vi "40G RF Switch Tool(NI 6509).vi"(4 "error in":errorcluster, 5 "Index":i8 min=0 max=100, 6 "arrayinput(1-48)":bool[][](array[boolean]), 7 "DAQ Device":enum16{"Dev1", "Dev2", "Dev3"}(ring)) -> ()   [LabVIEW 2011]
uses:
  <vilib>/Utility/error.llb/DialogType.ctl
  <vilib>/Utility/file.llb/Read From Spreadsheet File (I64).vi
  <vilib>/Utility/file.llb/Write To Spreadsheet File (I64).vi
panel:
  in  "Arrayinput":bool[][](array[boolean])=array80x96[7680 elements]
  in  "Tap":enum32{"P1-P5", "P6-P11"}(tab)
  in  "Index 3":i32[](array[numeric])=[1, 2, 3, 4, 5, 6, 7, 8, 9, 10, 11, 12, 13, 14, 15, 16, 17, 18, 19, 20, 21, 22, 23, 24, 25, 26, 27, 28, 29, 30, 31, 32, 33, 34, 35, 36, 37, 38, 39, 40, 41, 42, 43, 44, 45, 46, 47, 48, 49, 50, 51, 52, 53, 54, 55, 56, 57, 58, 59, 60, 61, 62, 63, 64, 65, 66, 67, 68, 69, 70, 71, 72, 73, 74, 75, 76, 77, 78, 79, 80]
  in  "PCI-6509: P0-P1-P2-P3-P4-P5":dbl[](array[numeric])=[0.0, 1.0, 2.0, 3.0, 4.0, 5.0, 6.0, 7.0, 0.0, 1.0, 2.0, 3.0, 4.0, 5.0, 6.0, 7.0, 0.0, 1.0, 2.0, 3.0, 4.0, 5.0, 6.0, 7.0, 0.0, 1.0, 2.0, 3.0, 4.0, 5.0, 6.0, 7.0, 0.0, 1.0, 2.0, 3.0, 4.0, 5.0, 6.0, 7.0, 0.0, 1.0, 2.0, 3.0, 4.0, 5.0, 6.0, 7.0]
  in  "Index 2":i32[](array[numeric])=[1, 2, 3, 4, 5, 6, 7, 8, 9, 10, 11, 12, 13, 14, 15, 16, 17, 18, 19, 20, 21, 22, 23, 24, 25, 26, 27, 28, 29, 30, 31, 32, 33, 34, 35, 36, 37, 38, 39, 40, 41, 42, 43, 44, 45, 46, 47, 48, 49, 50, 51, 52, 53, 54, 55, 56, 57, 58, 59, 60, 61, 62, 63, 64, 65, 66, 67, 68, 69, 70, 71, 72, 73, 74, 75, 76, 77, 78, 79, 80]
  in  "PCI-6509: P6-P7-P8-P9-P10-P11":dbl[](array[numeric])=[0.0, 1.0, 2.0, 3.0, 4.0, 5.0, 6.0, 7.0, 0.0, 1.0, 2.0, 3.0, 4.0, 5.0, 6.0, 7.0, 0.0, 1.0, 2.0, 3.0, 4.0, 5.0, 6.0, 7.0, 0.0, 1.0, 2.0, 3.0, 4.0, 5.0, 6.0, 7.0, 0.0, 1.0, 2.0, 3.0, 4.0, 5.0, 6.0, 7.0, 0.0, 1.0, 2.0, 3.0, 4.0, 5.0, 6.0, 7.0]
  in  "array input (49~96)":bool[][](array[boolean])
  in  "Switch Matrix":u16(ring)=4
  in  "Basic Path":path=path "D:/HPTS Development/VNA Automatic Data Save Tool 20151010(No DAQ)/Switch Matrix"
  out "Matrix List":string[](array[string])
  out "Path":path=path "D:/HPTS Development/VNA Automatic Data Save Tool 20151010(No DAQ)/Switch Matrix"
  in  "Modify":bool
  in  "Lines 4":tag="Dev3/port0/line0:7, Dev3/port1/line0:7, Dev3/port2/line0:7, Dev3/port3/line0:7, Dev3/port4/line0:7, Dev3/port5/line0:7, Dev3/port6/line0:7, Dev3/port7/line0:7, Dev3/port8/line0:7, Dev3/port9/line0:7, Dev3/port10/line0:7, Dev3/port11/line0:7" caption="Lines"
  in  "Lines 2":tag="Dev2/port0/line0:7, Dev2/port1/line0:7, Dev2/port2/line0:7, Dev2/port3/line0:7, Dev2/port4/line0:7, Dev2/port5/line0:7, Dev2/port6/line0:7, Dev2/port7/line0:7, Dev2/port8/line0:7, Dev2/port9/line0:7, Dev2/port10/line0:7, Dev2/port11/line0:7" caption="Lines"
  in  "Lines":tag="Dev1/port0/line0:7, Dev1/port1/line0:7, Dev1/port2/line0:7, Dev1/port3/line0:7, Dev1/port4/line0:7, Dev1/port5/line0:7, Dev1/port6/line0:7, Dev1/port7/line0:7, Dev1/port8/line0:7, Dev1/port9/line0:7, Dev1/port10/line0:7, Dev1/port11/line0:7"
  in  "name to assign":string="NI6509"
  # "RF Matrix Control System By NI PCI-6509 DAQmx Card"
  # "20151016"
  # "SW-04 A"
  # "SW01 & 02"
  # "SW-02 A"
  # "SW-03 A"
  # "SW-01 A"
  # "-------------P0------------"
  # "-------------P1------------"
  # "-------------P2------------"
  # "-------------P3------------"
  # "-------------P4------------"
  # "-------------P5------------"
  # "SW-01 B"
  # "SW-04 B"
  # "SW03 & SW04"
  # "SW-02 B"
  # "SW-03 B"
  # "-------------P6------------"
  # "-------------P7------------"
  # "-------------P8------------"
  # "------------P9------------"
  # "-------------P10----------"
  # "-------------P11-----------"
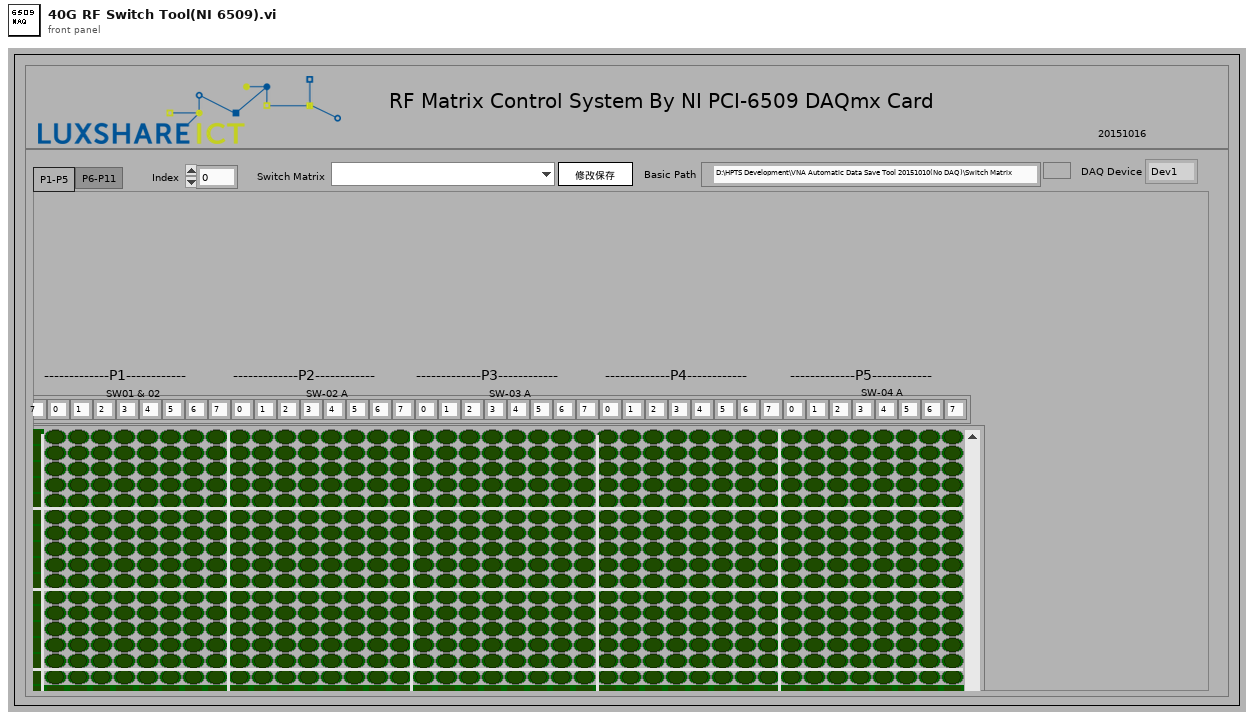
[diagram p1: front panel]
types:
  T1 = typedef "DialogType.ctl" = u16
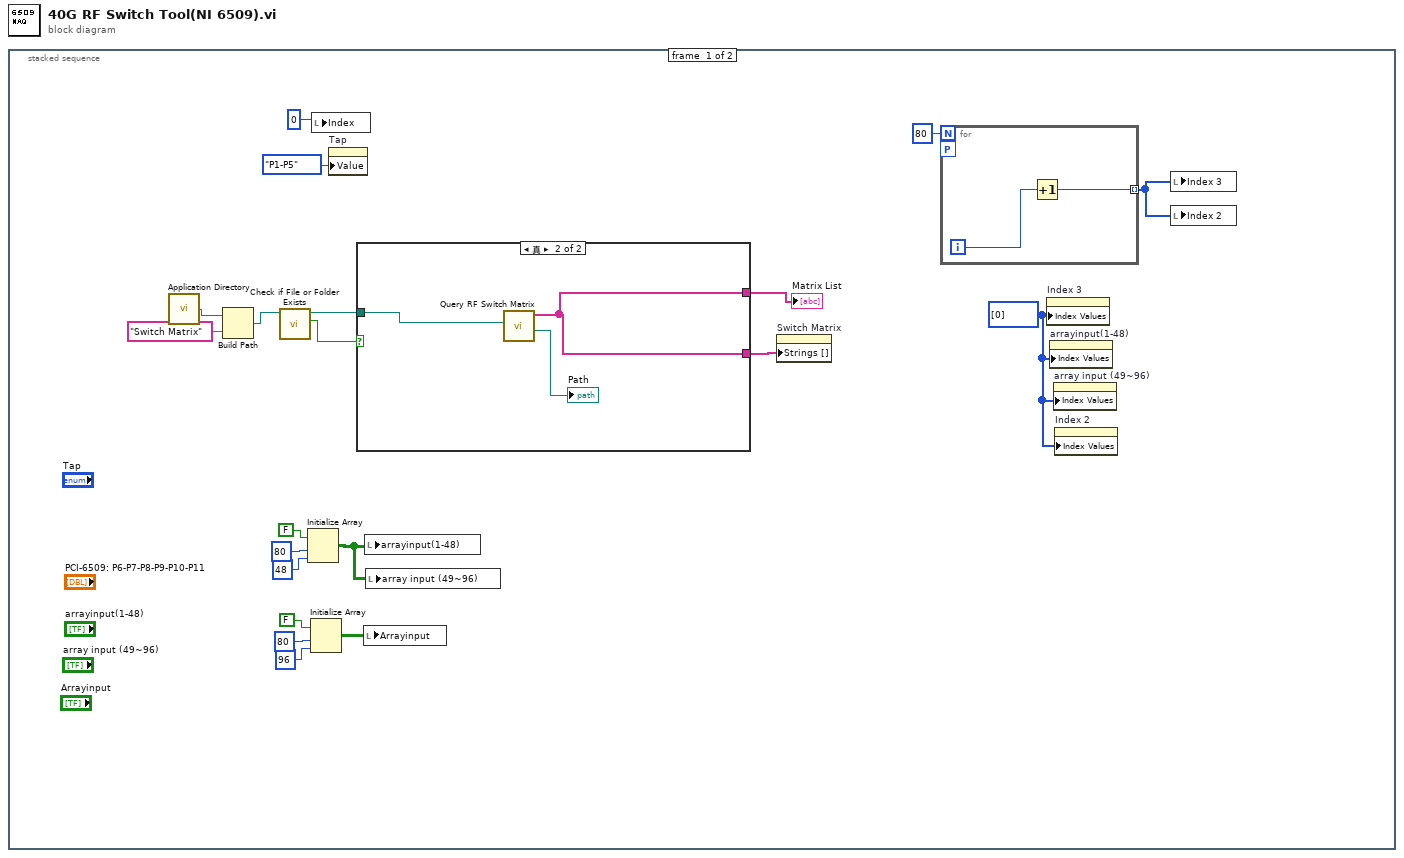
[diagram p0: block diagram]
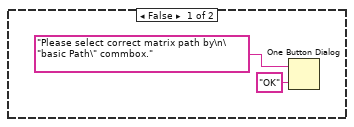
[diagram p2: hidden frame]
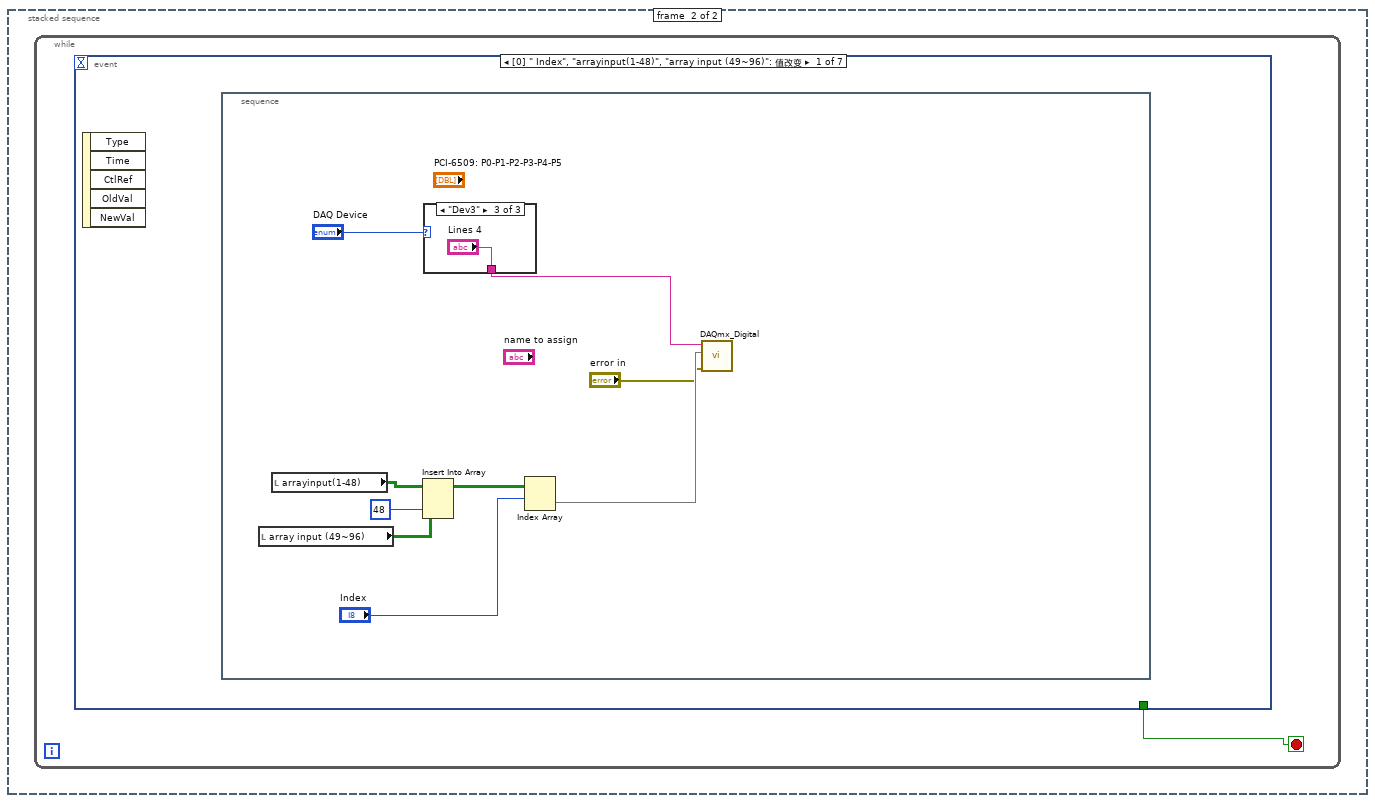
[diagram p3: hidden frame]
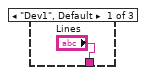
[diagram p4: hidden frame]
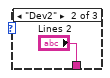
[diagram p5: hidden frame]
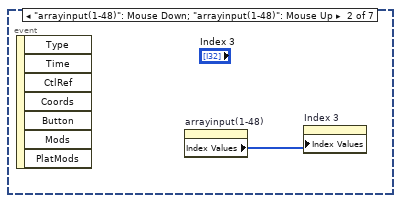
[diagram p6: hidden frame]
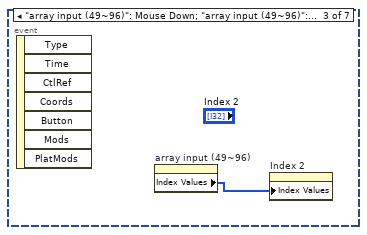
[diagram p7: hidden frame]
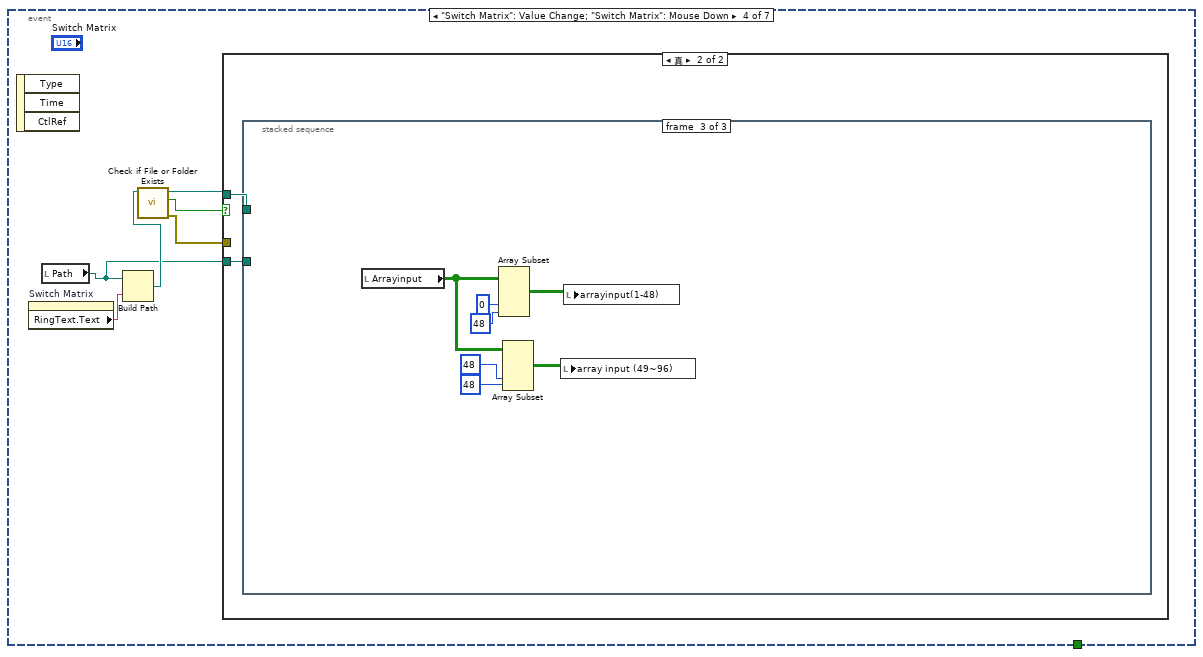
[diagram p8: hidden frame]
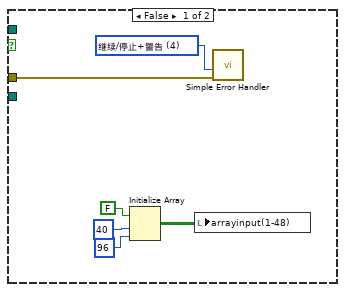
[diagram p9: hidden frame]
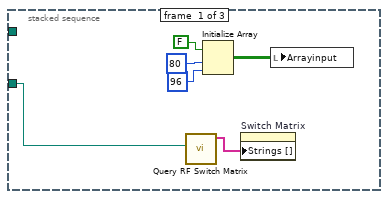
[diagram p10: hidden frame]
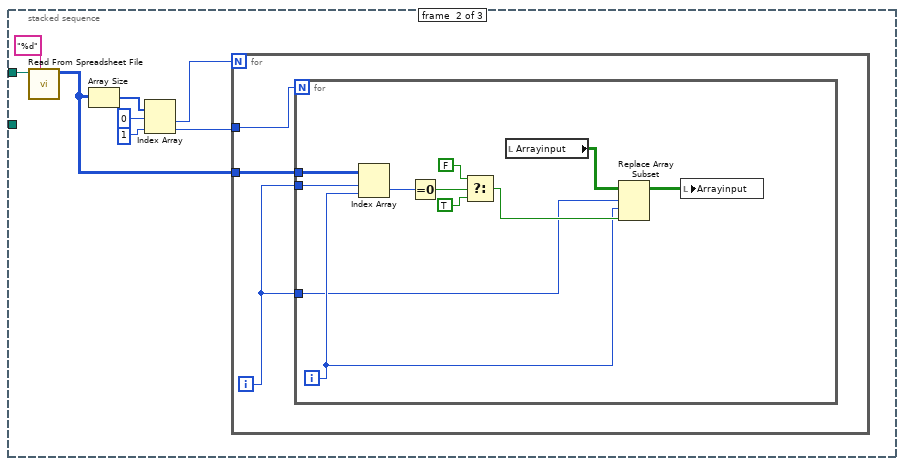
[diagram p11: hidden frame]
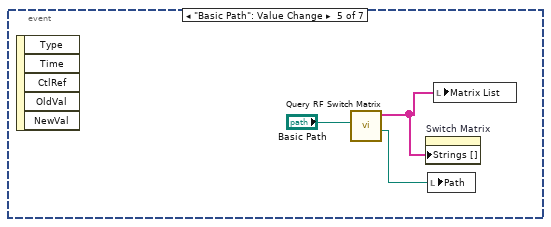
[diagram p12: hidden frame]
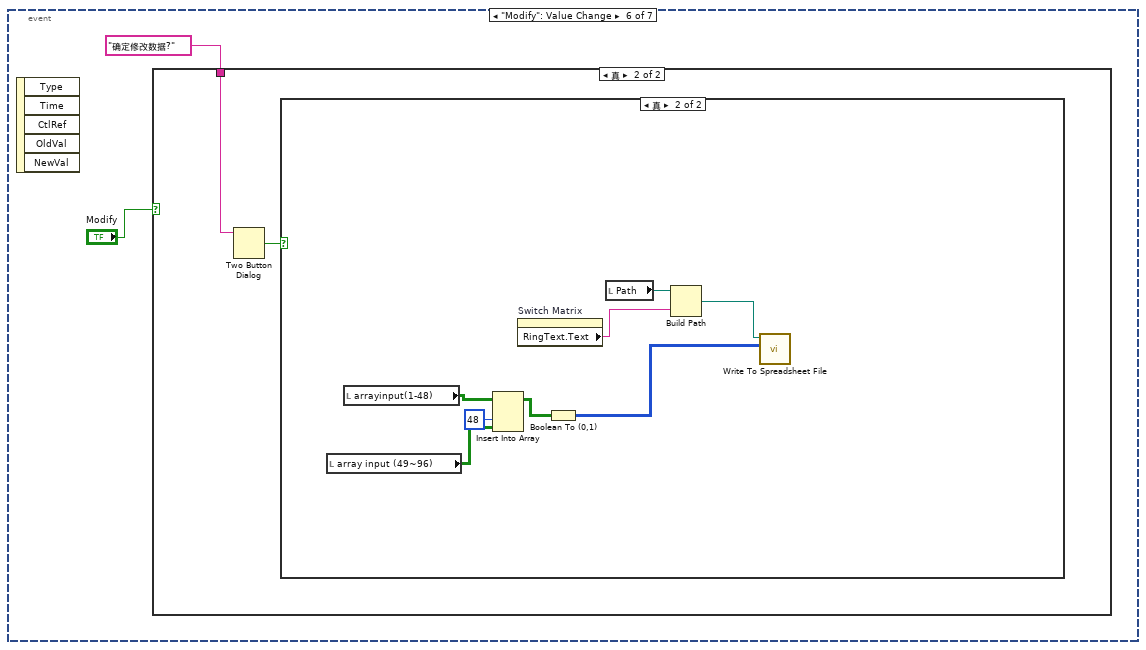
[diagram p13: hidden frame]
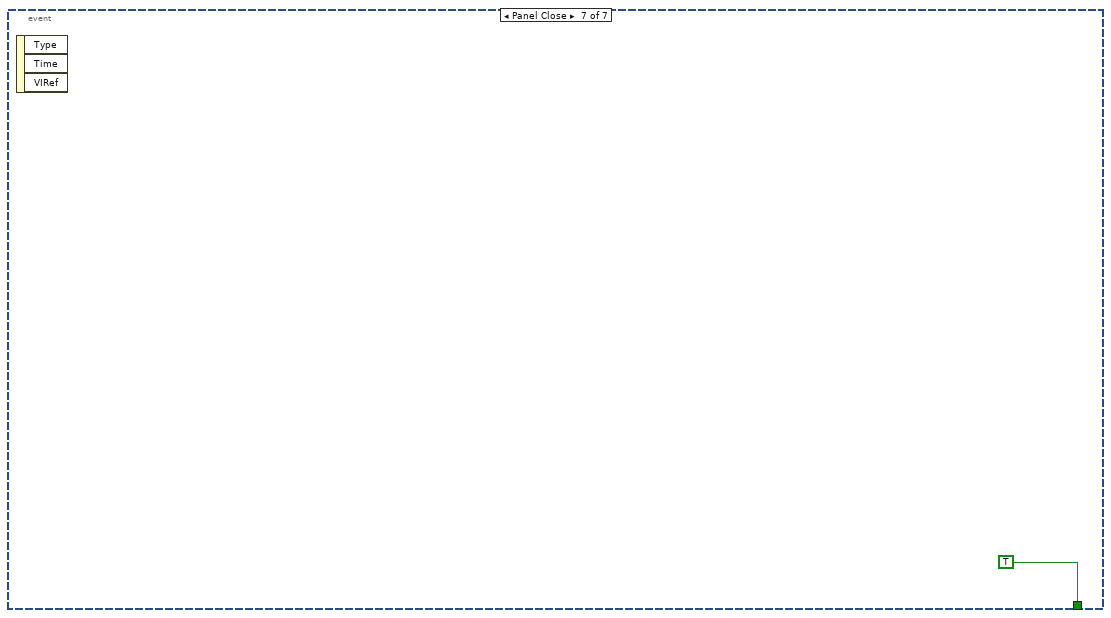
[diagram p16: hidden frame]
diagram:
  n1 = stacked-sequence {
    frame #0 {
      w2 = u32[] [0] ("索引值")
      n2 = call <vilib>:"Application Directory.vi"() -> ("Application Directory"=w19:path)
      n3 = Build Path(base path=w19, name or relative path="Switch Matrix" ("名称或相对路径")) -> (appended path=w17:path)
      n4 = call <vilib>:"Check if File or Folder Exists.vi"("path"=w17) -> ("file or folder exists?"=w16:bool, "dup path"=w15:path)  [unwired: 8 in, 1 out]
      n5 = Initialize Array(FALSE, 80 ("维数大小"), 48 ("维数大小")) -> (w8:bool[][])
      n6 = Initialize Array(FALSE, 80 ("维数大小"), 96 ("维数大小")) -> (w4:bool[][])
      n7 = local write "Index"(i8 0 ("Action Index)")) -> ()
      n8 = property on="Tap" class="TabCtl (严格)"("Value"=enum32{"P1-P5", "P6-P11"}."P1-P5" ("Tap")) -> ()  [unwired: 2 in, 2 out]
      n9 = case shown="真" w16 {
        tunnel: w15 -> [_ w26]
        tunnel: [_ w25] -> w14
        tunnel: [_ w25] -> w13
        frame False {
          n10 = One Button Dialog(message="Please select correct matrix path by\n\"basic Path\" commbox." ("消息"), button name ("OK")="OK" ("按钮名称（“确定”）")) -> ()  [unwired: 1 out]
        }
        frame True {
          n11 = call "Query RF Switch Matrix.vi"("Basic Path"=w26) -> ("Path"=→"Path":path, "Matrix List"=w25:string[])  [unwired: 9 in]
        }
      }
      "Matrix List" <- w14
      n12 = local write "Arrayinput"(w4) -> ()
      n13 = local write "arrayinput(1-48)"(w8) -> ()
      n14 = local write "array input (49~96)"(w8) -> ()
      n15 = property on="Switch Matrix" class="Ring (严格)"("Strings []"=w13) -> ()  [unwired: 2 in, 2 out]
      n16 = for "For循环" {
        N: 80 -> [_]
        tunnel: [w21] -> w3 mode=indexing
        workers-P: _ -> [_]
        i -> [w22]
        n17 = Increment(x=w22) -> (x+1=w21:i32)
      }
      n18 = property on="Index 3" class="Arr (严格)"("Index Values"=w2) -> ()  [unwired: 2 in, 2 out]
      n19 = property on="arrayinput(1-48)" class="Arr (严格)"("Index Values"=w2) -> ()  [unwired: 2 in, 2 out]
      n20 = property on="array input (49~96)" class="Arr (严格)"("Index Values"=w2) -> ()  [unwired: 2 in, 2 out]
      n21 = property on="Index 2" class="Arr (严格)"("Index Values"=w2) -> ()  [unwired: 2 in, 2 out]
      n22 = local write "Index 3"(w3) -> ()
      n23 = local write "Index 2"(w3) -> ()
    }
    frame #1 {
      n24 = while {
        stop <- w28 stop-if-true
        n25 = event shown="[0] \" Index\", \"arrayinput(1-48)\", \"array input (49~96)\": 值改变" {
          selector: _ -> [_ _ _ _ _ _ _]
          dyn-events: _ -> [_ _ _ _ _ _ _]
          timeout: _ -> [_ _ _ _ _ _ _]
          tunnel: [_ _ _ _ _ _ TRUE] -> w28
          event "Index", "arrayinput(1-48)", "array input (49~96)": Value Change {
            n26 = event-data() -> ()  [unwired: 1 in, 5 out]
            n27 = stacked-sequence {
              frame #0 {
                n28 = local read "array input (49~96)"() -> (w34:bool[][])
                n29 = local read "arrayinput(1-48)"() -> (w35:bool[][])
                n30 = Insert Into Array(array=w35, index (col)=48 ("禁用的索引 (列)"), new element=w34) -> (w33:bool[][])  [unwired: 1 in]
                n31 = case shown="\"Dev3\"" "DAQ Device" {
                  tunnel: ["Lines" "Lines 2" "Lines 4"] -> w31
                  frame "Dev1", Default {
                  }
                  frame "Dev2" {
                  }
                  frame "Dev3" {
                  }
                }
                n32 = Index Array(array=w33, index (row)="Index") -> (element=w30:bool[])  [unwired: 1 in]
                n33 = call "DAQmx_Digital.vi"("Error in"="error in", "Data"=w30, "lines"=w31) -> ()  [unwired: 8 in, 1 out]
              }
            }
          }
          event "arrayinput(1-48)": Mouse Down; "arrayinput(1-48)": Mouse Up {
            n34 = event-data() -> ()  [unwired: 1 in, 7 out]
            n35 = property on="arrayinput(1-48)" class="Arr (严格)"() -> ("Index Values"=w41:u32[])  [unwired: 2 in, 2 out]
            n36 = property on="Index 3" class="Arr (严格)"("Index Values"=w41) -> ()  [unwired: 2 in, 2 out]
          }
          event "array input (49~96)": Mouse Down; "array input (49~96)": Mouse Up {
            n37 = event-data() -> ()  [unwired: 1 in, 7 out]
            n38 = property on="array input (49~96)" class="Arr (严格)"() -> ("Index Values"=w42:u32[])  [unwired: 2 in, 2 out]
            n39 = property on="Index 2" class="Arr (严格)"("Index Values"=w42) -> ()  [unwired: 2 in, 2 out]
          }
          event "Switch Matrix": Value Change; "Switch Matrix": Mouse Down {
            n40 = event-data() -> ()  [unwired: 1 in, 3 out]
            n41 = property on="Switch Matrix" class="Ring (严格)"() -> ("RingText.Text"=w48:string)  [unwired: 2 in, 2 out]
            n42 = local read "Path"() -> (w43:path)
            n43 = Build Path(base path=w43, name or relative path=w48) -> (appended path=w47:path)
            n44 = call <vilib>:"Check if File or Folder Exists.vi"("path"=w47) -> ("error out"=w46:errorcluster, "file or folder exists?"=w45:bool, "dup path"=w44:path)  [unwired: 8 in]
            n45 = case shown="真" w45 {
              tunnel: w46 -> [w54 _]
              tunnel: w44 -> [_ w56]
              tunnel: w43 -> [_ w55]
              frame False {
                w53 = T1 4 items=["无对话框", "确定信息", "继续或停止信息", "确定信息＋警告", "继续/停止+警告"] ("type of dialog (OK msg:1)")
                n46 = Initialize Array(FALSE, 40 ("维数大小"), 96 ("维数大小")) -> (w49:bool[][])
                n47 = local write "arrayinput(1-48)"(w49) -> ()
                n48 = call <vilib>:"Simple Error Handler.vi"("type of dialog (OK msg:1)"=w53, "error in (no error)"=w54) -> ()  [unwired: 3 in, 5 out]
              }
              frame True {
                n49 = stacked-sequence {
                  tunnel: w56 -> [_ w63 _]
                  tunnel: w55 -> [w59 _ _]
                  frame #0 {
                    n50 = call "Query RF Switch Matrix.vi"("Basic Path"=w59) -> ("Matrix List"=w58:string[])  [unwired: 9 in, 1 out]
                    n51 = Initialize Array(FALSE, 80 ("维数大小"), 96 ("维数大小")) -> (w57:bool[][])
                    n52 = property on="Switch Matrix" class="Ring (严格)"("Strings []"=w58) -> ()  [unwired: 2 in, 2 out]
                    n53 = local write "Arrayinput"(w57) -> ()
                  }
                  frame #1 {
                    n54 = call-poly <vilib>:"Read From Spreadsheet File.vi"("format (%d)"="%d" ("format (%.3f)"), "file path (dialog if empty)"=w63) -> ("all rows"=w70:i64[][])  [unwired: 5 in, 4 out]
                    n55 = Array Size(array=w70) -> (size(s)=w64:i32[])
                    n56 = Index Array(array=w64, index #1=0 ("索引"), index #2=1 ("索引")) -> (element #1=w67:i32, element #2=w68:i32)
                    n57 = for "For循环" {
                      N: w67 -> [_]
                      tunnel: w68 -> [w73]
                      tunnel: w70 -> [w72]
                      i -> [w71]
                      n58 = for "For循环" {
                        N: w73 -> [_]
                        tunnel: w72 -> [w84]
                        tunnel: w71 -> [w83]
                        tunnel: w71 -> [w76]
                        i -> [w77]
                        n59 = Index Array(array=w84, index (row)=w83, index (col)=w77) -> (element=w82:i64)
                        n60 = Equal To 0?(x=w82) -> (x = 0?=w81:bool)
                        n61 = Select(t=FALSE, s=w81, f=TRUE) -> (s? t:f=w78:bool)
                        n62 = local read "Arrayinput"() -> (w75:bool[][])
                        n63 = Replace Array Subset(array=w75, new element=w78, index (row)=w76, index (col)=w77) -> (w74:bool[][])
                        n64 = local write "Arrayinput"(w74) -> ()
                      }
                    }
                  }
                  frame #2 {
                    n65 = local read "Arrayinput"() -> (w89:bool[][])
                    n66 = Array Subset(array=w89, index (col)=0 ("索引"), length (col)=48 ("长度")) -> (w86:bool[][])  [unwired: 2 in]
                    n67 = Array Subset(array=w89, index (col)=48 ("索引"), length (col)=48 ("长度")) -> (w85:bool[][])  [unwired: 2 in]
                    n68 = local write "array input (49~96)"(w85) -> ()
                    n69 = local write "arrayinput(1-48)"(w86) -> ()
                  }
                }
              }
            }
          }
          event "Basic Path": Value Change {
            n70 = event-data() -> ()  [unwired: 1 in, 5 out]
            n71 = call "Query RF Switch Matrix.vi"("Basic Path"="Basic Path") -> ("Path"=w93:path, "Matrix List"=w94:string[])  [unwired: 9 in]
            n72 = property on="Switch Matrix" class="Ring (严格)"("Strings []"=w94) -> ()  [unwired: 2 in, 2 out]
            n73 = local write "Path"(w93) -> ()
            n74 = local write "Matrix List"(w94) -> ()
          }
          event "Modify": Value Change {
            n75 = event-data() -> ()  [unwired: 1 in, 5 out]
            n76 = case shown="真" "Modify" {
              tunnel: "确定修改数据?" ("消息") -> [_ w98]
              frame False {
              }
              frame True {
                n77 = Two Button Dialog(message=w98) -> (T button?=w97:bool)  [unwired: 2 in]
                n78 = case shown="真" w97 {
                  frame False {
                  }
                  frame True {
                    n79 = local read "array input (49~96)"() -> (w101:bool[][])
                    n80 = local read "arrayinput(1-48)"() -> (w102:bool[][])
                    n81 = Insert Into Array(array=w102, index (col)=48 ("禁用的索引 (列)"), new element=w101) -> (w100:bool[][])  [unwired: 1 in]
                    n82 = property on="Switch Matrix" class="Ring (严格)"() -> ("RingText.Text"=w103:string)  [unwired: 2 in, 2 out]
                    n83 = Boolean To (0,1)(Boolean=w100) -> (0, 1=w106:i16[][])
                    n84 = local read "Path"() -> (w104:path)
                    n85 = Build Path(base path=w104, name or relative path=w103) -> (appended path=w105:path)
                    n86 = call-poly <vilib>:"Write To Spreadsheet File.vi"("2D data"=w106, "file path (dialog if empty)"=w105) -> ()  [unwired: 6 in, 1 out]
                  }
                }
              }
            }
          }
          event Panel Close {
            n87 = event-data() -> ()  [unwired: 1 in, 3 out]
          }
        }
      }
    }
  }
